vi "MGI Wrap String to Character Width.vi"(1 "Wrap length(Characters)":i32, 2 "Unwrapped string":string) -> (0 "Wrapped String":string)   [LabVIEW 2020]
doc: "Use line feeds to perform word wrap i.e. no line can be longer than the specified length. Line feeds overwrite spaces or are inserted into very long words.\n\nAuthored by David A. Moore\nsupport@mooregoodideas.com\nwww.mooregoodideas.com\n\nCopyright (c) 2010, Moore Good Ideas, Inc.\n\nAll rights reserved.\n\nRedistribution and use in source and binary forms, with or without modification, are permitted provided that the following conditions are met:\n\n * Redistributions of source code must retain the above copyright notice, this list of conditions and the following disclaimer.\n * Redistributions in binary form must reproduce the above copyright notice, this list of conditions and the following disclaimer in the documentation and/or other materials provided with the distribution.\n * Neither the name of Moore Good Ideas, Inc. nor the names of its contributors may be used to endorse or promote products derived from this software without specific prior written permission.\n\nTHIS SOFTWARE IS PROVIDED BY THE COPYRIGHT HOLDERS AND CONTRIBUTORS \"AS IS\" AND ANY EXPRESS OR IMPLIED WARRANTIES, INCLUDING, BUT NOT LIMITED TO, THE IMPLIED WARRANTIES OF MERCHANTABILITY AND FITNESS FOR A PARTICULAR PURPOSE ARE DISCLAIMED. IN NO EVENT SHALL THE COPYRIGHT OWNER OR CONTRIBUTORS BE LIABLE FOR ANY DIRECT, INDIRECT, INCIDENTAL, SPECIAL, EXEMPLARY, OR CONSEQUENTIAL DAMAGES (INCLUDING, BUT NOT LIMITED TO, PROCUREMENT OF SUBSTITUTE GOODS OR SERVICES; LOSS OF USE, DATA, OR PROFITS; OR BUSINESS INTERRUPTION) HOWEVER CAUSED AND ON ANY THEORY OF LIABILITY, WHETHER IN CONTRACT, STRICT LIABILITY, OR TORT (INCLUDING NEGLIGENCE OR OTHERWISE) ARISING IN ANY WAY OUT OF THE USE OF THIS SOFTWARE, EVEN IF ADVISED OF THE POSSIBILITY OF SUCH DAMAGE."
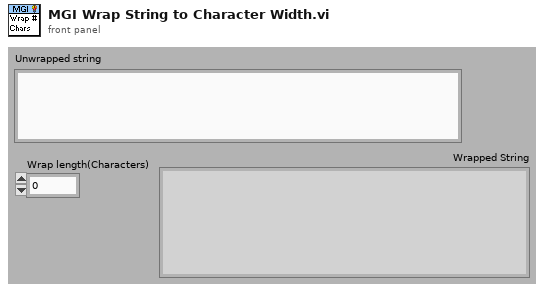
[diagram p1: front panel]
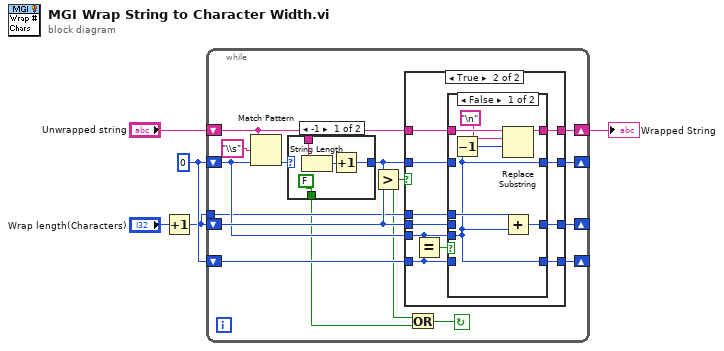
[diagram p0: block diagram]
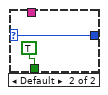
[diagram p2: hidden frame]
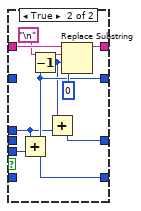
[diagram p4: hidden frame]
diagram:
  w4 = 0
  n1 = Increment(x="Wrap length(Characters)") -> (x+1=w3:i32)
  n2 = while {
    shift-right: [w19] -> w1
    shift-left: "Unwrapped string" -> [w13]
    shift-right: [w18] -> _
    shift-left: w4 -> [w10]
    shift-right: [w16] -> _
    shift-left: w3 -> [w17]
    shift-right: [w11] -> _
    shift-left: w4 -> [w12]
    tunnel: w3 -> [w9]
    stop <- w6 continue-if-true
    n3 = Match Pattern(string=w13, regular expression="\\s", offset (0)=w10) -> (offset past match=w15:i32)  [unwired: 3 out]
    n4 = case shown="-1" w15 {
      selector: w15 -> [_ w26]
      tunnel: [w21 w26] -> w14
      tunnel: w13 -> [w24 _]
      tunnel: [FALSE TRUE] -> w7
      frame -1 {
        n5 = String Length(string=w24) -> (length=w22:i32)
        n6 = Increment(x=w22) -> (x+1=w21:i32)
      }
      frame Default {
      }
    }
    n7 = Greater?(x=w14, y=w17) -> (0:w8:bool)
    n8 = case shown="True" w8 {
      tunnel: w14 -> [w29 w37]
      tunnel: w13 -> [w30 w36]
      tunnel: [w30 w35] -> w19
      tunnel: [w29 w31] -> w18
      tunnel: w17 -> [w28 w38]
      tunnel: [w28 w32] -> w16
      tunnel: w10 -> [_ w40]
      tunnel: w12 -> [w27 w39]
      tunnel: [w27 w34] -> w11
      tunnel: w9 -> [_ w33]
      frame False {
      }
      frame True {
        n9 = Equal?(x=w40, y=w39) -> (x = y?=w41:bool)
        n10 = case shown="False" w41 {
          tunnel: w40 -> [w42 w53]
          tunnel: w39 -> [_ _]
          tunnel: w38 -> [_ _]
          tunnel: w37 -> [_ _]
          tunnel: w36 -> [w48 w57]
          tunnel: [w45 w56] -> w35
          tunnel: [w42 w52] -> w34
          tunnel: w33 -> [w44 w51]
          tunnel: [w43 w49] -> w32
          tunnel: [w42 w52] -> w31
          frame False {
            n11 = Decrement(x=w42) -> (x-1=w47:i32)
            n12 = Replace Substring(3:w47, 4:"\n", 5:w48) -> (1:w45:string)  [unwired: 1 in, 1 out]
            n13 = Add(x=w44, y=w42) -> (x+y=w43:i32)
          }
          frame True {
            n14 = Add(x=w51, y=w53) -> (x+y=w52:i32)
            n15 = Decrement(x=w52) -> (x-1=w50:i32)
            n16 = Add(x=w50, y=w51) -> (x+y=w49:i32)
            n17 = Replace Substring(2:0 ("length (len. of substring)"), 3:w50, 4:"\n", 5:w57) -> (1:w56:string)  [unwired: 1 out]
          }
        }
      }
    }
    n18 = Or(x=w8, y=w7) -> (x .or. y?=w6:bool)
  }
  "Wrapped String" <- w1
